vi "总磷数据时间处理.vi"(10 "总氮测量数据区":T1 {"单位" items=["ug/L", "mg/L", "ppm", "mg/m3", "cm", "ppb", "ug/m3", "%", "nmol/mol", "umol/mol", "MPN/L", "MPN/100ml", "ng/m3", "NTU", "无量纲", "ms/cm", "us/cm", "℃", "mV", "万个/L"]}, 11 "总磷测量数据区":T1 {"单位" items=["ug/L", "mg/L", "ppm", "mg/m3", "cm", "ppb", "ug/m3", "%", "nmol/mol", "umol/mol", "MPN/L", "MPN/100ml", "ng/m3", "NTU", "无量纲", "ms/cm", "us/cm", "℃", "mV", "万个/L"]}) -> (3 "总磷测量数据区 2":T1 {"单位" items=["ug/L", "mg/L", "ppm", "mg/m3", "cm", "ppb", "ug/m3", "%", "nmol/mol", "umol/mol", "MPN/L", "MPN/100ml", "ng/m3", "NTU", "无量纲", "ms/cm", "us/cm", "℃", "mV", "万个/L"]})   [LabVIEW 2016, in "斯坦道仪器.lvlib"]
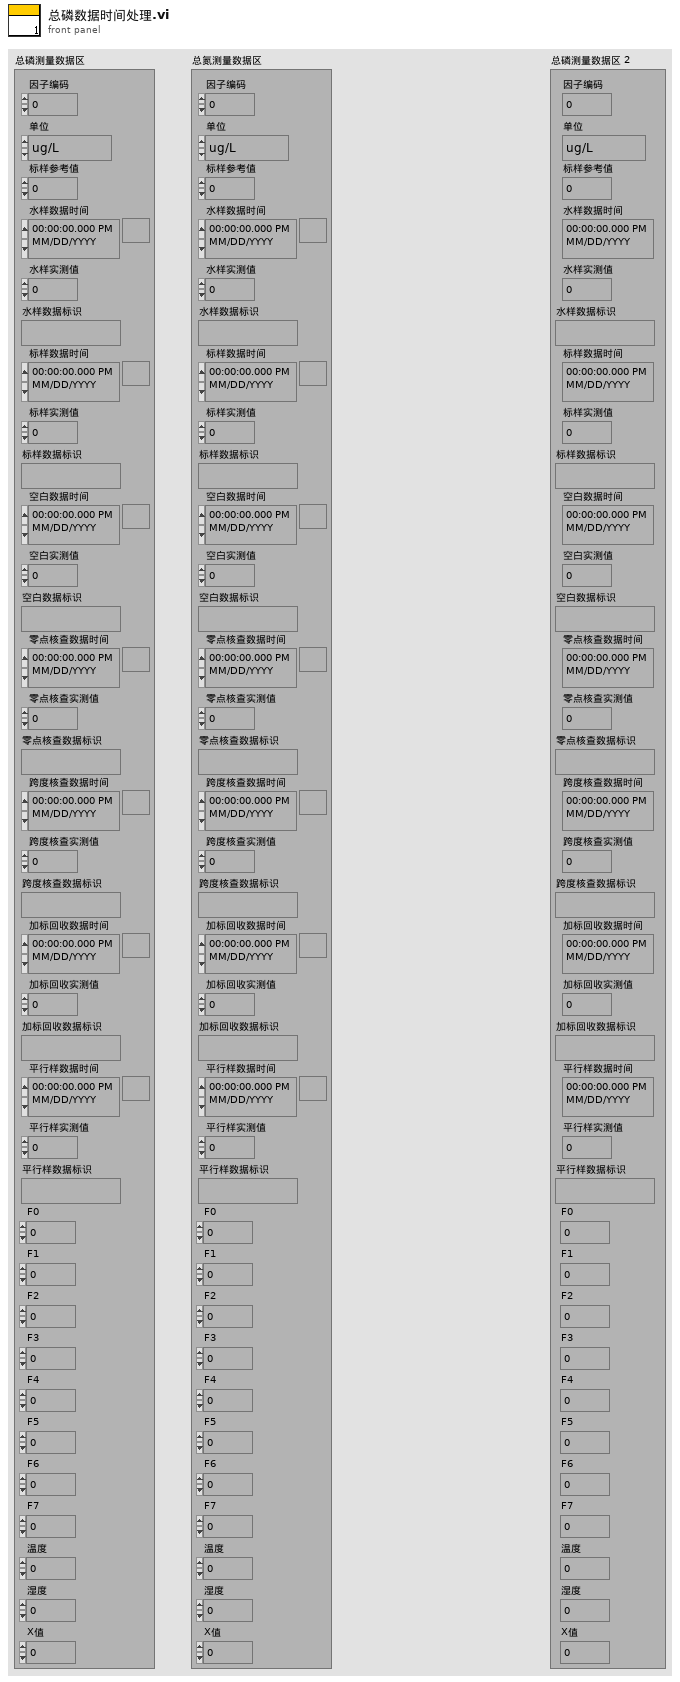
[diagram p1: front panel]
types:
  T1 = cluster{"因子编码":u32, "单位":u16, "标样参考值":sgl, "水样数据时间":timestamp, "水样实测值":sgl, "水样数据标识":string, "标样数据时间":timestamp, "标样实测值":sgl, "标样数据标识":string, "空白数据时间":timestamp, "空白实测值":sgl, "空白数据标识":string, "零点核查数据时间":timestamp, "零点核查实测值":sgl, "零点核查数据标识":string, "跨度核查数据时间":timestamp, "跨度核查实测值":sgl, "跨度核查数据标识":string, "加标回收数据时间":timestamp, "加标回收实测值":sgl, "加标回收数据标识":string, "平行样数据时间":timestamp, "平行样实测值":sgl, "平行样数据标识":string, "F0":sgl, "F1":sgl, "F2":sgl, "F3":sgl, "F4":sgl, "F5":sgl, "F6":sgl, "F7":sgl, "温度":sgl, "湿度":sgl, "X值":sgl}
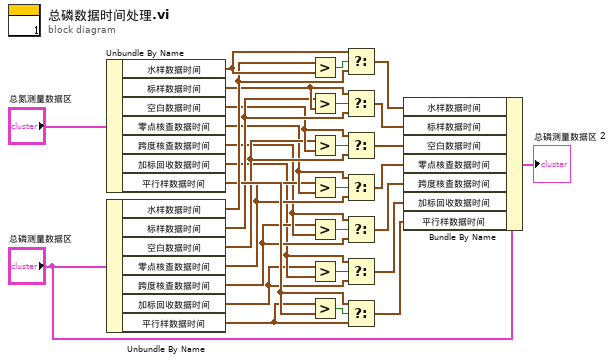
[diagram p0: block diagram]
diagram:
  n1 = Unbundle By Name("总氮测量数据区") -> ("水样数据时间"=w27:timestamp, "标样数据时间"=w15:timestamp, "空白数据时间"=w12:timestamp, "零点核查数据时间"=w9:timestamp, "跨度核查数据时间"=w6:timestamp, "加标回收数据时间"=w2:timestamp, "平行样数据时间"=w23:timestamp)
  n2 = Unbundle By Name("总磷测量数据区") -> ("水样数据时间"=w26:timestamp, "标样数据时间"=w14:timestamp, "空白数据时间"=w11:timestamp, "零点核查数据时间"=w8:timestamp, "跨度核查数据时间"=w5:timestamp, "加标回收数据时间"=w1:timestamp, "平行样数据时间"=w22:timestamp)
  n3 = Greater?(x=w26, y=w27) -> (0:w28:bool)
  n4 = Greater?(x=w14, y=w15) -> (0:w16:bool)
  n5 = Greater?(x=w11, y=w12) -> (0:w17:bool)
  n6 = Greater?(x=w8, y=w9) -> (0:w18:bool)
  n7 = Greater?(x=w5, y=w6) -> (0:w19:bool)
  n8 = Greater?(x=w1, y=w2) -> (0:w20:bool)
  n9 = Greater?(x=w22, y=w23) -> (0:w24:bool)
  n10 = Select(t=w27, s=w28, f=w26) -> (s? t:f=w25:timestamp)
  n11 = Select(t=w15, s=w16, f=w14) -> (s? t:f=w13:timestamp)
  n12 = Select(t=w12, s=w17, f=w11) -> (s? t:f=w10:timestamp)
  n13 = Select(t=w9, s=w18, f=w8) -> (s? t:f=w7:timestamp)
  n14 = Select(t=w6, s=w19, f=w5) -> (s? t:f=w4:timestamp)
  n15 = Select(t=w2, s=w20, f=w1) -> (s? t:f=w3:timestamp)
  n16 = Select(t=w23, s=w24, f=w22) -> (s? t:f=w21:timestamp)
  n17 = Bundle By Name(cluster="总磷测量数据区", "水样数据时间"=w25, "标样数据时间"=w13, "空白数据时间"=w10, "零点核查数据时间"=w7, "跨度核查数据时间"=w4, "加标回收数据时间"=w3, "平行样数据时间"=w21) -> (→"总磷测量数据区 2":T1)
